vi "Close.vi"(8 "error in (no error)":errorcluster, 11 "Data in":refnum<class "Var Bus.lvclass">) -> (0 "error out":errorcluster, 3 "Data out":refnum<class "Var Bus.lvclass">)   [LabVIEW 2021, in "Var Bus.lvclass"]
uses:
  Var Bus.lvclass
  Data Classes/Source/Abs_Types/Type/Abs_Type.lvclass
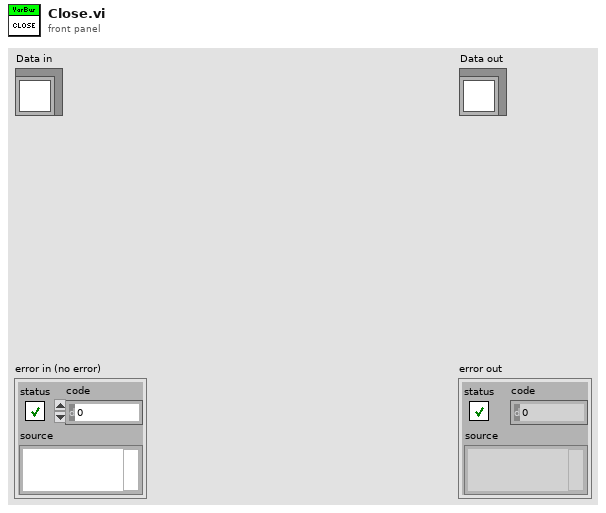
[diagram p1: front panel]
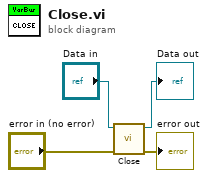
[diagram p0: block diagram]
diagram:
  n1 = call-parent "Close.vi"("error in (no error)"="error in (no error)", "Data in"="Data in") -> ("error out"=→"error out":errorcluster, "Data out"=→"Data out":refnum<class "Var Bus.lvclass">)  [unwired: 8 in]
